vi "Local_Path_New (SubVI).vi"(0 "x_lat_arr":dbl[](array[numeric]), 2 "WP no_pre":i32, 5 "y_long_arr":dbl[](array[numeric]), 7 "vel_arr":dbl[](array[numeric]), 9 "x_lat_c":dbl, 11 "y_long_c":dbl, 13 "# of pnt":i32) -> (4 "INDEX(Near Point)":i32, 8 "Lat(Local)":dbl[](array[numeric]), 10 "Long(Local)":dbl[](array[numeric]), 15 "Vel(Local)":dbl[](array[numeric]))   [LabVIEW 2020]
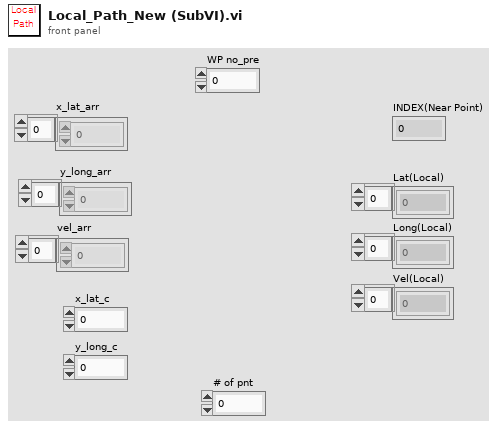
[diagram p1: front panel]
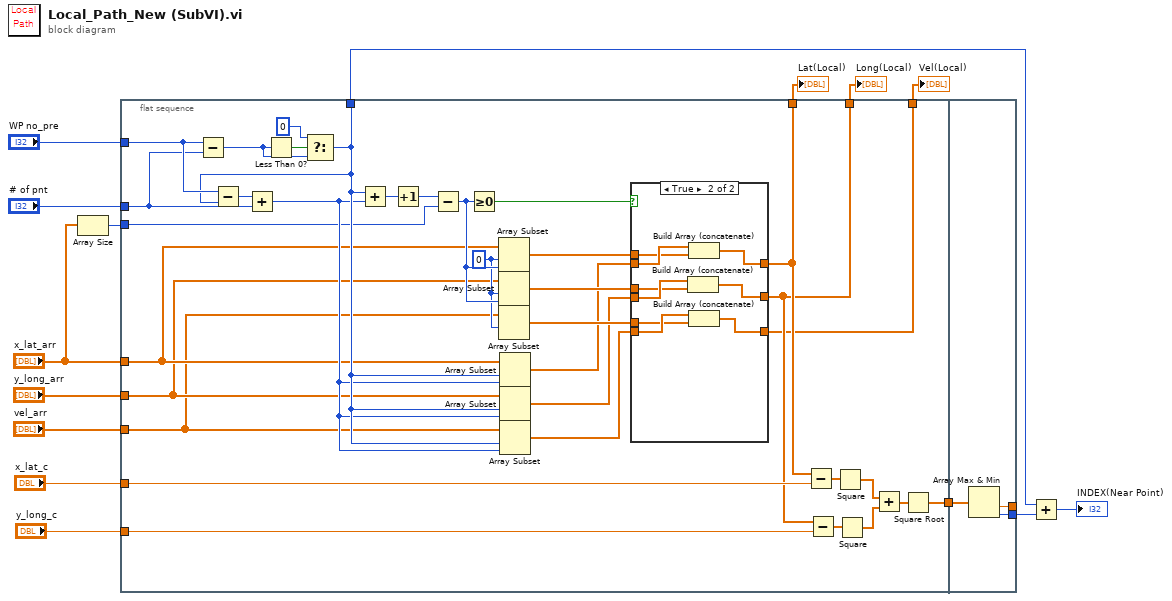
[diagram p0: block diagram]
diagram:
  n1 = Array Size(array="x_lat_arr") -> (size(s)=w4:i32)
  n2 = flat-sequence {
    tunnel: "WP no_pre" -> [w45]
    tunnel: "# of pnt" -> [w44]
    tunnel: "x_lat_arr" -> [w28]
    tunnel: "y_long_arr" -> [w27]
    tunnel: "x_lat_c" -> [w38]
    tunnel: "y_long_c" -> [w37]
    tunnel: [w36] -> w10
    tunnel: [w35] -> w8
    tunnel: "vel_arr" -> [w26]
    tunnel: w4 -> [w31]
    tunnel: [w18] -> w3
    tunnel: [w17] -> w2
    tunnel: [w16] -> w1
    tunnel: w10 -> [w64]
    tunnel: [w63] -> _
    tunnel: [w62] -> w9
    frame #0 {
      w29 = 0 ("인덱스")
      n3 = Subtract(x=w45, y=w44) -> (x-y=w48:i32)
      n4 = Less Than 0?(x=w48) -> (x < 0?=w49:bool)
      n5 = Select(t=0, s=w49, f=w48) -> (s? t:f=w35:i32)
      n6 = Subtract(x=w45, y=w35) -> (x-y=w47:i32)
      n7 = Add(x=w47, y=w44) -> (x+y=w34:i32)
      n8 = Add(x=w35, y=w34) -> (x+y=w33:i32)
      n9 = Increment(x=w33) -> (x+1=w32:i32)
      n10 = Subtract(x=w32, y=w31) -> (x-y=w30:i32)
      n11 = Greater Or Equal To 0?(x=w30) -> (x >= 0?=w25:bool)
      n12 = Array Subset(array=w28, index=w29, length=w30) -> (w24:dbl[])
      n13 = Array Subset(array=w27, index=w29, length=w30) -> (w23:dbl[])
      n14 = Array Subset(array=w26, index=w29) -> (w22:dbl[])  [unwired: 1 in]
      n15 = Array Subset(array=w28, index=w35, length=w34) -> (w19:dbl[])
      n16 = Array Subset(array=w27, index=w35, length=w34) -> (w20:dbl[])
      n17 = Array Subset(array=w26, index=w35, length=w34) -> (w21:dbl[])
      n18 = case shown="True" w25 {
        tunnel: w19 -> [w52 w61]
        tunnel: w24 -> [_ w60]
        tunnel: w23 -> [_ w53]
        tunnel: w20 -> [w51 w54]
        tunnel: [w52 w59] -> w18
        tunnel: [w51 w58] -> w17
        tunnel: w21 -> [w50 w57]
        tunnel: w22 -> [_ w56]
        tunnel: [w50 w55] -> w16
        frame False {
        }
        frame True {
          n19 = Build Array (concatenate)(w54, w53) -> (w58:dbl[])
          n20 = Build Array (concatenate)(w61, w60) -> (w59:dbl[])
          n21 = Build Array (concatenate)(w57, w56) -> (w55:dbl[])
        }
      }
      n22 = Subtract(x=w18, y=w38) -> (x-y=w43:dbl[])
      n23 = Subtract(x=w17, y=w37) -> (x-y=w42:dbl[])
      n24 = Square(x=w43) -> (x^2=w41:dbl[])
      n25 = Square(x=w42) -> (x^2=w40:dbl[])
      n26 = Add(x=w41, y=w40) -> (x+y=w39:dbl[])
      n27 = Square Root(x=w39) -> (sqrt(x)=w36:dbl[])
    }
    frame #1 {
      n28 = Array Max & Min(array=w64) -> (min value=w63:dbl, min index (indices)=w62:i32)  [unwired: 2 out]
    }
  }
  n29 = Add(x=w8, y=w9) -> (x+y=→"INDEX(Near Point)":i32)
  "Lat(Local)" <- w3
  "Long(Local)" <- w2
  "Vel(Local)" <- w1
